vi "Double to Xcontrol converter.vi"(9 "Parameter Impuls Series":T1 {"Gain" format="%.1f"; "Offset" format="%.1f"}, 10 "No Impulses":i32, 11 "Impulses":dbl[][](array[numeric])) -> (3 "Array":T2(array[cluster]))   [LabVIEW 2013]
uses:
  src/core/type-defs/TD_Impulse Parameter.ctl
  src/core/core.lvlib
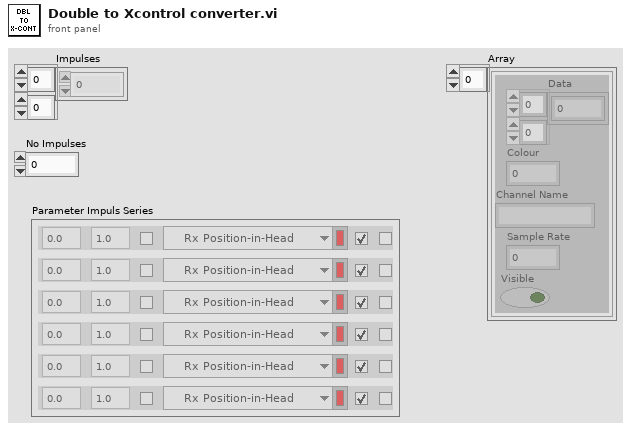
[diagram p1: front panel]
types:
  T1 = typedef "core.lvlib/TD_Impulse Parameter.ctl" = cluster{"Color":u32, "Visible":bool, "Channel":u16, "Invert":bool, "Desaccade":bool, "Offset":dbl, "Gain":dbl}[]
  T2 = cluster{"Data":dbl[][], "Colour":u32, "Channel Name":string, "Sample Rate":dbl, "Visible":bool}[]
  T3 = cluster{"Data":dbl[][], "Colour":u32, "Channel Name":string, "Sample Rate":dbl, "Visible":bool}
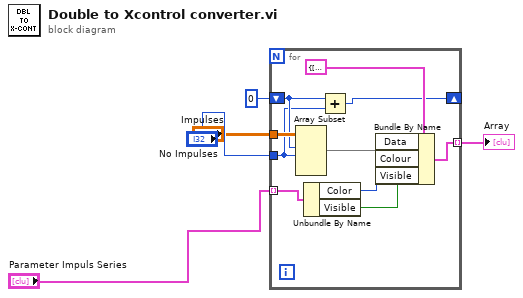
[diagram p0: block diagram]
diagram:
  n1 = for {
    tunnel: "Impulses" -> [w15]
    tunnel: "No Impulses" -> [w7]
    tunnel: "Parameter Impuls Series" -> [w11] mode=indexing
    tunnel: [w13] -> w5 mode=indexing
    shift-right: [w6] -> _
    shift-left: 0 -> [w8]
    n2 = Array Subset(array=w15, index (row)=w8, length (row)=w7) -> (w12:dbl[][])  [unwired: 2 in]
    n3 = Unbundle By Name(w11) -> ("Color"=w10:u32, "Visible"=w9:bool)
    n4 = Add(x=w8, y=w7) -> (x+y=w6:i32)
    n5 = Bundle By Name(cluster=T3 {"Data"=[[1.0, 2.0, 3.0, 4.0, 5.0]], "Colour"=255, "Channel Name"="test1", "Sample Rate"=0.0, "Visible"=TRUE} ("Cluster"), "Data"=w12, "Colour"=w10, "Visible"=w9) -> (w13:T3)
  }
  "Array" <- w5
